vi "Get Async FIFO Refs.vi"(8 "error in (no error)":errorcluster, 10 "Data Access API In":refnum<class "Data Access Engine.lvclass">, 11 "Async State Vars In":T1) -> (0 "error out":errorcluster, 2 "Data Access API Out":refnum<class "Data Access Engine.lvclass">, 3 "Async State Vars Out":T1)   [LabVIEW 2020, in "Waveform-Processing-Custom-Device Engine.lvlib"]
uses:
  Waveform-Processing-Custom-Device Engine.lvlib
  Types/AsyncStateVariables.ctl
  <vilib>/NI VeriStand/Custom Device Waveform API/Single Waveform Read (DBL)/Single Waveform Read (DBL).lvclass
  <vilib>/NI VeriStand/Custom Device Waveform API/Single Waveform Write (DBL)/Single Waveform Write (DBL).lvclass
  <vilib>/NI VeriStand/Custom Device API/Waveform Data Reference.ctl
  <vilib>/NI/NIVS Inline Async API/_Data Access Engine/Data Access Engine/Types/Write.DVR.ctl
  <vilib>/NI/NIVS Inline Async API/_Data Access Engine/Access Type Classes/Write/Write.lvclass
  <vilib>/NI/NIVS Inline Async API/_Data Access Engine/Data Access Engine/Types/Read.DVR.ctl
  <vilib>/NI/NIVS Inline Async API/_Data Access Engine/Access Type Classes/Read/Read.lvclass
  <vilib>/NI/NIVS Inline Async API/_Data Access Engine/Data Access Engine/Data Access Engine.lvclass
  Shared/Constants.vi
  <vilib>/NI/NIVS Inline Async API/_Data Access Engine/Data Access Engine/Methods/Read.Lookup.vi
  <vilib>/NI/NIVS Inline Async API/_Data Access Engine/Data Access Engine/Methods/Write.Lookup.vi
  Shared/Waveform-Processing-Custom-Device Shared.lvlib
  <vilib>/NI VeriStand/Custom Device API/Custom Device API.lvlib
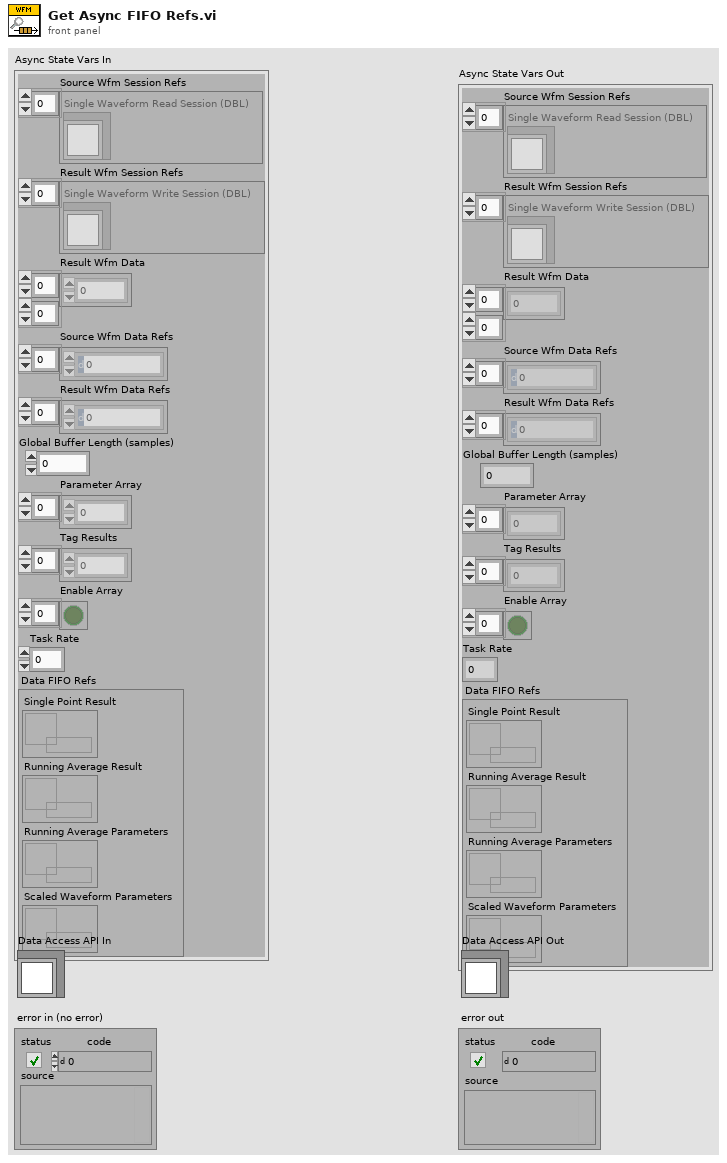
[diagram p1: front panel]
types:
  T1 = typedef "Waveform-Processing-Custom-Device Engine.lvlib/AsyncStateVariables.ctl" = cluster{"Source Wfm Session Refs":refnum<class "Single Waveform Read (DBL).lvclass">[], "Result Wfm Session Refs":refnum<class "Single Waveform Write (DBL).lvclass">[], "Result Wfm Data":dbl[][], "Source Wfm Data Refs":T2[], "Result Wfm Data Refs":T2[], "Global Buffer Length (samples)":dbl, "Parameter Array":dbl[], "Tag Results":dbl[], "Enable Array":bool[], "Task Rate":dbl, "Data FIFO Refs":cluster{"Single Point Result":T3, "Running Average Result":T3, "Running Average Parameters":T4, "Scaled Waveform Parameters":T4}}
  T2 = typedef "Custom Device API.lvlib/Waveform Data Reference.ctl" = i32
  T3 = typedef "Data Access Engine.lvlib/Data Access Engine.lvclass/Write.DVR.ctl" = refnum<data-value>
  T4 = typedef "Data Access Engine.lvlib/Data Access Engine.lvclass/Read.DVR.ctl" = refnum<data-value>
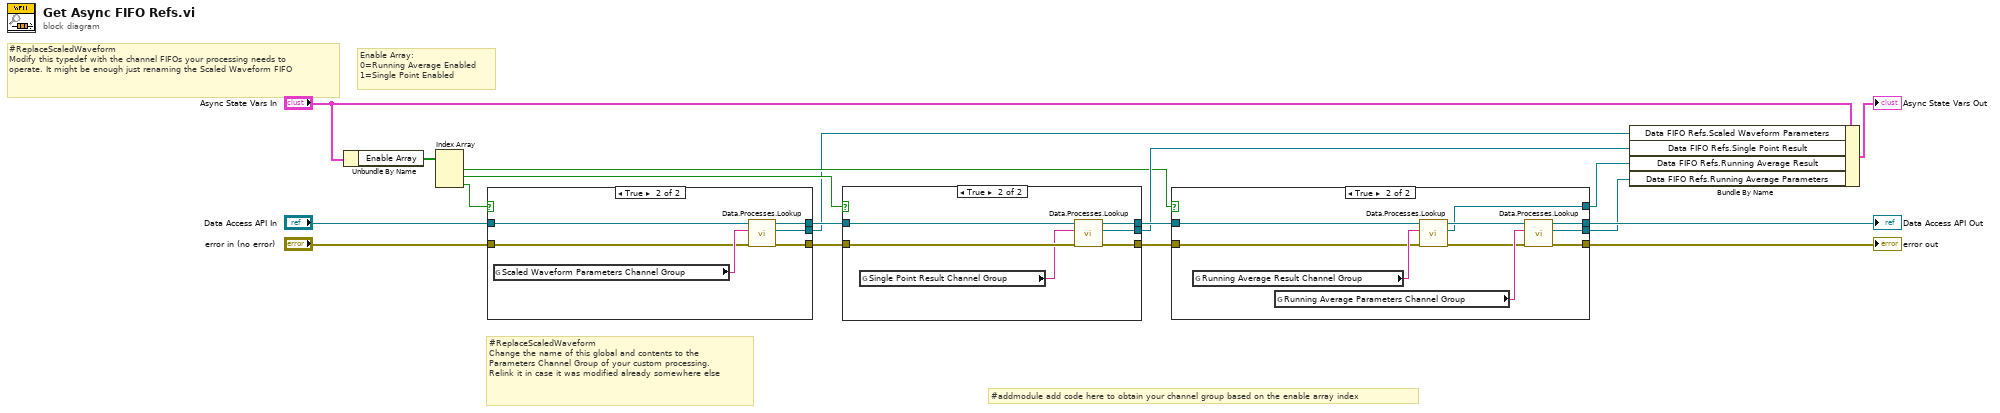
[diagram p0: block diagram]
diagram:
  # "#ReplaceScaledWaveform \nModify this typedef with the channel FIFOs your processing needs to\noperate. It might be enough just renaming the Scaled Waveform FIFO"
  # "#ReplaceScaledWaveform \nChange the name of this global and contents to the\nParameters Channel Group of your custom processing.\nRelink it in case it was modified already somewhere else"
  # "#addmodule add code here to obtain your channel group based on the enable array index"
  # "Enable Array:\n0=Running Average Enabled\n1=Single Point Enabled"
  n1 = Unbundle By Name("Async State Vars In") -> ("Enable Array"=w11:bool[])
  n2 = Index Array(array=w11) -> (element #1=w7:bool, element #2=w10:bool, element #3=w2:bool)  [unwired: 3 in]
  n3 = case shown="True" w2 {
    tunnel: [w19 w26] -> w5
    tunnel: "Data Access API In" -> [w19 w21]
    tunnel: [_ w25] -> w1
    tunnel: [w20 w23] -> w6
    tunnel: "error in (no error)" -> [w20 w22]
    frame False {
    }
    frame True {
      n4 = global read "Constants.vi" "Scaled Waveform Parameters Channel Group"() -> (w24:string)
      n5 = call-poly <vilib>:"Data.Processes.Lookup.vi"("error in (no error)"=w22, "Name"=w24, "Data Access API in"=w21) -> ("error out"=w23:errorcluster, "Ref"=w25:T4, "Data Access API out"=w26:refnum<class "Data Access Engine.lvclass">)  [unwired: 5 in, 1 out]
    }
  }
  n6 = case shown="True" w10 {
    tunnel: w5 -> [w28 w34]
    tunnel: [w28 w33] -> w16
    tunnel: w6 -> [w27 w32]
    tunnel: [_ w31] -> w14
    tunnel: [w27 w29] -> w9
    frame False {
      # "If single point is not enabled, pass data through\nand create default refnum for FIFO"
    }
    frame True {
      n7 = global read "Constants.vi" "Single Point Result Channel Group"() -> (w30:string)
      n8 = call-poly <vilib>:"Data.Processes.Lookup.vi"("error in (no error)"=w32, "Name"=w30, "Data Access API in"=w34) -> ("error out"=w29:errorcluster, "Ref"=w31:T3, "Data Access API out"=w33:refnum<class "Data Access Engine.lvclass">)  [unwired: 5 in, 1 out]
    }
  }
  n9 = case shown="True" w7 {
    tunnel: [w35 w45] -> w18
    tunnel: w16 -> [w35 w44]
    tunnel: [_ w43] -> w15
    tunnel: [w36 w39] -> w13
    tunnel: w9 -> [w36 w38]
    tunnel: [_ w37] -> w8
    frame False {
      # "If running average is not enabled, pass data through\nand create default refnum for both FIFOs"
    }
    frame True {
      n10 = global read "Constants.vi" "Running Average Result Channel Group"() -> (w42:string)
      n11 = global read "Constants.vi" "Running Average Parameters Channel Group"() -> (w41:string)
      n12 = call-poly <vilib>:"Data.Processes.Lookup.vi"("error in (no error)"=w38, "Name"=w42, "Data Access API in"=w44) -> ("error out"=w40:errorcluster, "Ref"=w37:T3, "Data Access API out"=w46:refnum<class "Data Access Engine.lvclass">)  [unwired: 5 in, 1 out]
      n13 = call-poly <vilib>:"Data.Processes.Lookup.vi"("error in (no error)"=w40, "Name"=w41, "Data Access API in"=w46) -> ("error out"=w39:errorcluster, "Ref"=w43:T4, "Data Access API out"=w45:refnum<class "Data Access Engine.lvclass">)  [unwired: 5 in, 1 out]
    }
  }
  "error out" <- w13
  "Data Access API Out" <- w18
  n14 = Bundle By Name(cluster="Async State Vars In", "Data FIFO Refs.Scaled Waveform Parameters"=w1, "Data FIFO Refs.Single Point Result"=w14, "Data FIFO Refs.Running Average Result"=w8, "Data FIFO Refs.Running Average Parameters"=w15) -> (→"Async State Vars Out":T1)
